vi "ClusterToVars.vi"(0 "Cluster XY":cluster{dbl[], dbl[]}) -> (1 "R value":dbl, 2 "Fi value":dbl)   [LabVIEW 2020]
doc: "Creates spherical coordinates by given X and Y."
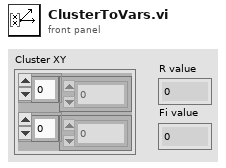
[diagram p1: front panel]
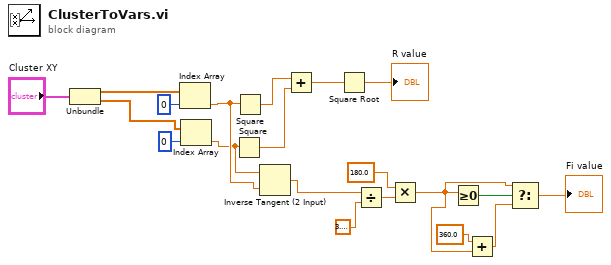
[diagram p0: block diagram]
diagram:
  n1 = Unbundle("Cluster XY") -> (w17:dbl[], w20:dbl[])
  n2 = Index Array(array=w17, index=0) -> (element=w3:dbl)
  n3 = Index Array(array=w20, index=0) -> (element=w2:dbl)
  n4 = Square(x=w2) -> (x^2=w4:dbl)
  n5 = Square(x=w3) -> (x^2=w15:dbl)
  n6 = Inverse Tangent (2 Input)(1:w3, 2:w2) -> (0:w1:dbl)
  n7 = Add(x=w15, y=w4) -> (x+y=w14:dbl)
  n8 = Square Root(x=w14) -> (sqrt(x)=→"R value":dbl)
  n9 = Divide(x=w1, y=3.141592653589793) -> (x/y=w7:dbl)
  n10 = Multiply(x=180.0, y=w7) -> (x*y=w5:dbl)
  n11 = Greater Or Equal To 0?(x=w5) -> (x >= 0?=w12:bool)
  n12 = Add(x=360.0 ("y"), y=w5) -> (x+y=w11:dbl)
  n13 = Select(t=w5, s=w12, f=w11) -> (s? t:f=→"Fi value":dbl)
